vi "data_headers_subVI_w_gases.vi"(8 "Experiment Notes":string, 10 "Sample names":T1={"QCM1 sample name"="aQCM2", "QCM2 sample name"="aQCM2", "QCM3 sample name"="aQCM3", "QCM4 sample name"="aQCM4", "QCM5 sample name"="aQCM5", "QCM6 sample name"="aQCM6", "SRS sample name"="sample_SRS", "Keithley 2420 sample name"="Keithley2420", "Keithley 6430 sample name"="Keithley6430", "Keithley 2100 sample name"="Keithley6430", "Gas"="aQCM2", "Vapor"="aQCM2"}) -> (2 "data headers":string[](array[string]))   [LabVIEW 2014]
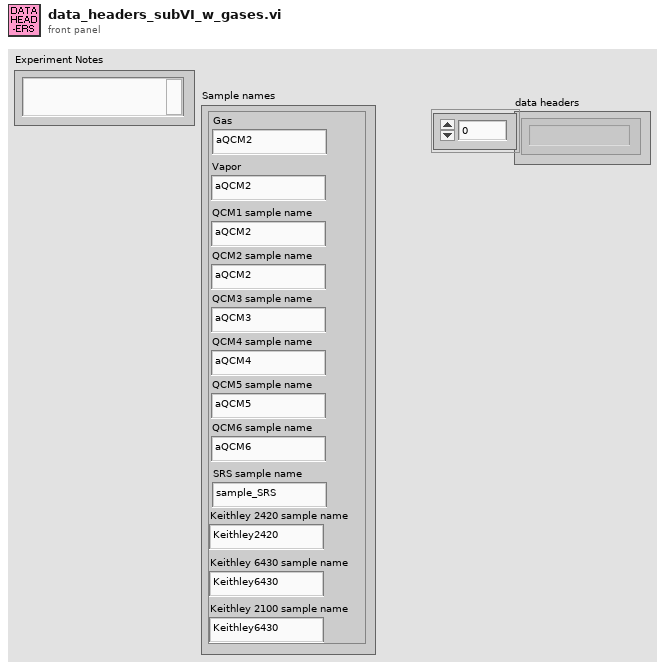
[diagram p1: front panel]
types:
  T1 = cluster{"QCM1 sample name":string, "QCM2 sample name":string, "QCM3 sample name":string, "QCM4 sample name":string, "QCM5 sample name":string, "QCM6 sample name":string, "SRS sample name":string, "Keithley 2420 sample name":string, "Keithley 6430 sample name":string, "Keithley 2100 sample name":string, "Gas":string, "Vapor":string}
  T2 = cluster{string, string, string, string, string, string}
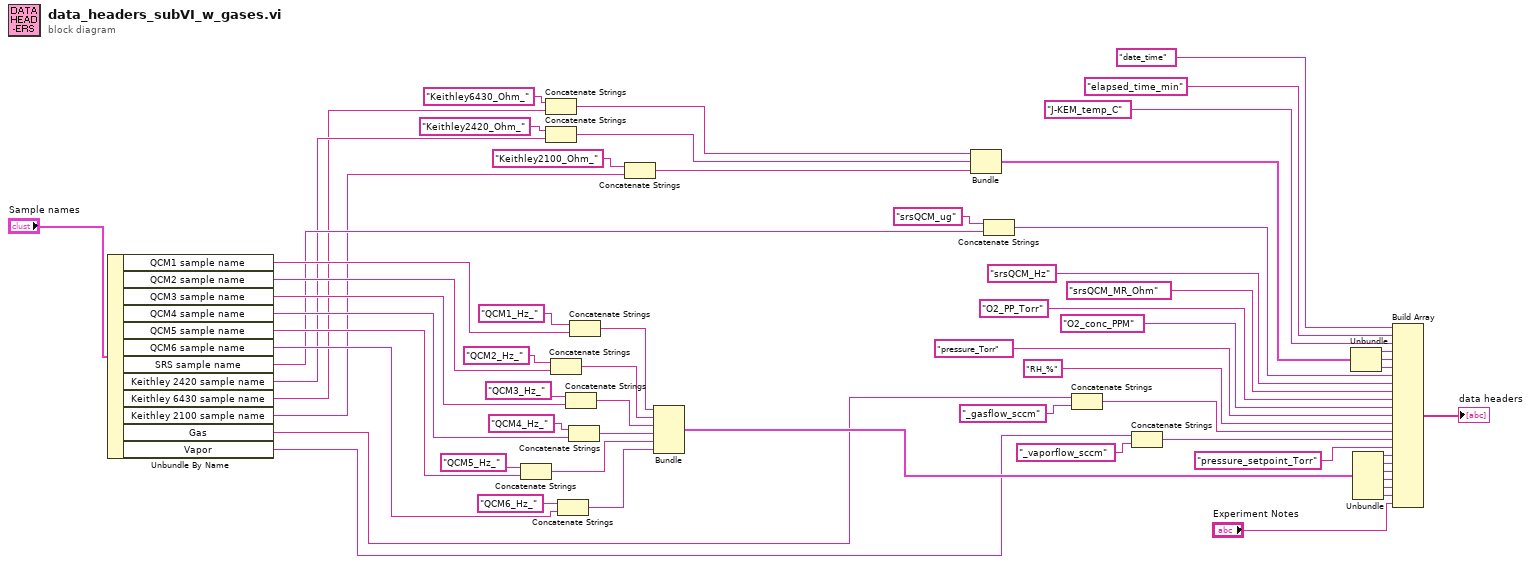
[diagram p0: block diagram]
diagram:
  n1 = Unbundle By Name("Sample names") -> ("QCM1 sample name"=w47:string, "QCM2 sample name"=w44:string, "QCM3 sample name"=w42:string, "QCM4 sample name"=w40:string, "QCM5 sample name"=w37:string, "QCM6 sample name"=w36:string, "SRS sample name"=w33:string, "Keithley 2420 sample name"=w32:string, "Keithley 6430 sample name"=w31:string, "Keithley 2100 sample name"=w29:string, "Gas"=w2:string, "Vapor"=w1:string)
  n2 = Concatenate Strings("QCM5_Hz_" ("string"), w37) -> (w16:string)
  n3 = Concatenate Strings("Keithley6430_Ohm_", w31) -> (w27:string)
  n4 = Concatenate Strings("Keithley2420_Ohm_" ("element"), w32) -> (w26:string)
  n5 = Concatenate Strings("QCM2_Hz_" ("string"), w44) -> (w19:string)
  n6 = Concatenate Strings("QCM6_Hz_" ("string"), w36) -> (w15:string)
  n7 = Concatenate Strings("QCM3_Hz_" ("string"), w42) -> (w18:string)
  n8 = Concatenate Strings("QCM4_Hz_" ("string"), w40) -> (w17:string)
  n9 = Concatenate Strings("QCM1_Hz_" ("string"), w47) -> (w20:string)
  n10 = Concatenate Strings("Keithley2100_Ohm_" ("element"), w29) -> (w25:string)
  n11 = Bundle(w20, w19, w18, w17, w16, w15) -> (w14:T2)  [unwired: 1 in]
  n12 = Bundle(w27, w26, w25) -> (w24:cluster{string, string, string})  [unwired: 1 in]
  n13 = Concatenate Strings("srsQCM_ug", w33) -> (w34:string)
  n14 = Concatenate Strings(w2, "_gasflow_sccm" ("element")) -> (w6:string)
  n15 = Concatenate Strings(w1, "_vaporflow_sccm" ("element")) -> (w5:string)
  n16 = Unbundle(w24) -> (w23:string, w22:string, w21:string)
  n17 = Unbundle(w14) -> (w8:string, w13:string, w12:string, w11:string, w10:string, w9:string)
  n18 = Build Array("date_time", "elapsed_time_min", "J-KEM_temp_C", w23, w22, w21, w34, "srsQCM_Hz", "srsQCM_MR_Ohm", "O2_PP_Torr" ("element"), "O2_conc_PPM" ("element"), "pressure_Torr" ("element"), "RH_%" ("element"), w6, w5, "pressure_setpoint_Torr" ("element"), w8, w13, w12, w11, w10, w9, "Experiment Notes") -> (→"data headers":string[])
